vi "load_handlers.vi"(11 "Handlers":string[](array[string])) -> (0 "Array":errorcluster[](array[cluster]), 3 "Handler refnums":refnum<vi>[](array[refnum]))   [LabVIEW 2011]
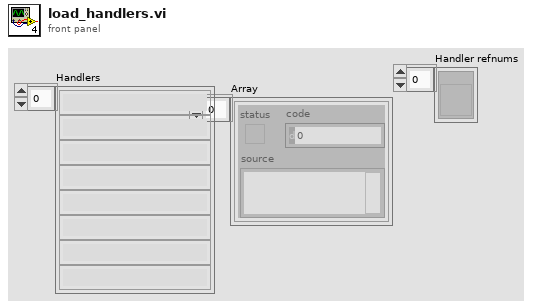
[diagram p1: front panel]
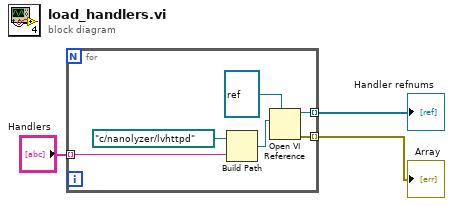
[diagram p0: block diagram]
diagram:
  n1 = for {
    tunnel: "Handlers" -> [w6] mode=indexing
    tunnel: [w8] -> w1 mode=indexing
    tunnel: [w7] -> w3 mode=indexing
    n2 = Build Path(base path=path "c:/nanolyzer/lvhttpd", name or relative path=w6) -> (appended path=w5:path)
    n3 = Open VI Reference(type specifier VI Refnum (for type only)=refnum<vi> refnum, vi path=w5) -> (vi reference=w8:refnum<vi>, error out=w7:errorcluster)  [unwired: 4 in]
  }
  "Array" <- w3
  "Handler refnums" <- w1
